vi "Remove Topic.vi"(8 "error in (no error)":errorcluster, 10 "Topic":refnum<class "Topic.lvclass">, 11 "TopicLookupTable":refnum<data-value>) -> (0 "error out":errorcluster, 3 "TopicLookupTable":refnum<data-value>)   [LabVIEW 2017, in "Mediator.lvlib" / "TopicLookupTable.lvclass"]
doc: "<License>\nCopyright © 2017 Composed Systems, LLC | All rights reserved\nwww.composed.io\n\nAuthor: Ethan Stern <ethan.stern@composed.io>\n\nThis software is provided \"AS IS\" WITHOUT WARRANTIES, either express or implied, AND IS FOR EDUCATIONAL PURPOSES ONLY.\n</License>"
uses:
  TopicLookupTable.lvclass
  Topic/Topic.lvclass
  C:/Program Files (x86)/National Instruments/LabVIEW 2017/vi.lib/ActorFramework/Actor/Actor.lvclass
  TopicLookupTable.lvclass/TopicLookupTable.ctl
  <vilib>/ActorFramework/Actor/Actor.lvclass/Actor.ctl
  <vilib>/ActorFramework/Message Enqueuer/Message Enqueuer.lvclass/Message Enqueuer.ctl
  Topic/Topic.lvclass/Topic.ctl
  <vilib>/ActorFramework/Message Enqueuer/Message Enqueuer.lvclass
  <vilib>/ActorFramework/Actor/Read Self Enqueuer.vi
  <vilib>/ActorFramework/Message Enqueuer/Init from Existing Queue.vi
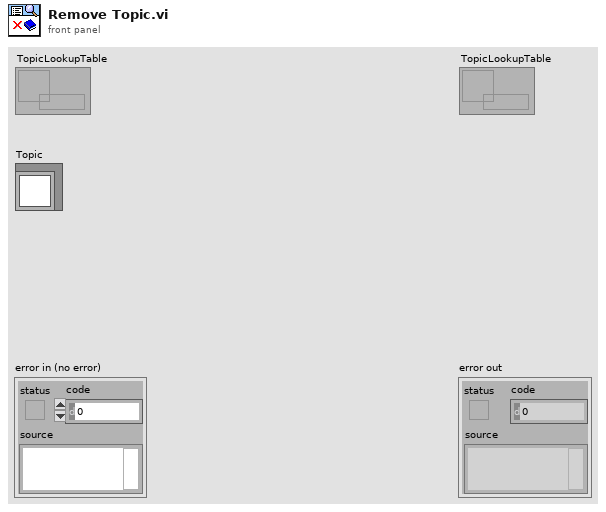
[diagram p1: front panel]
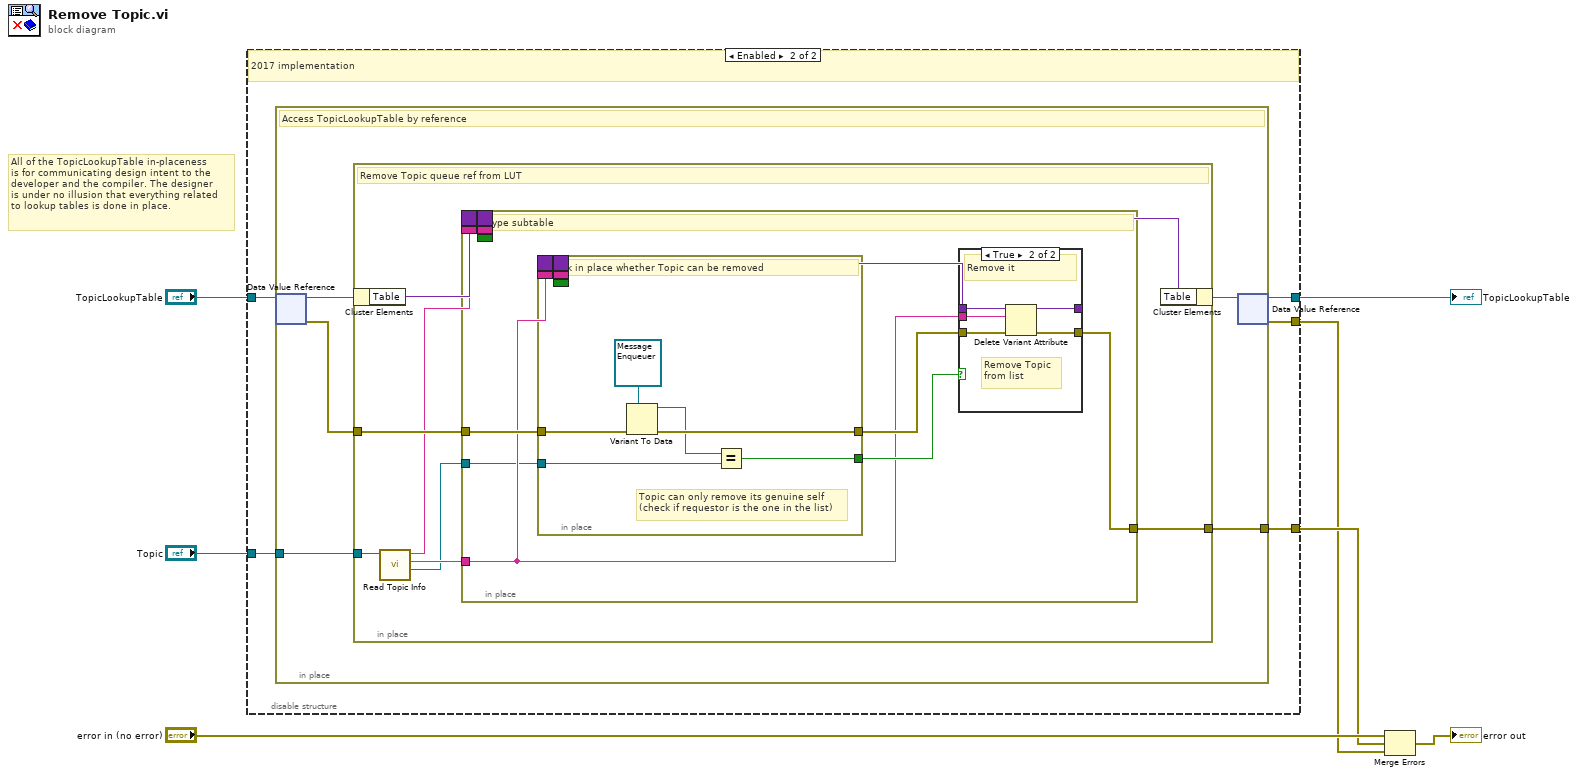
[diagram p0: block diagram]
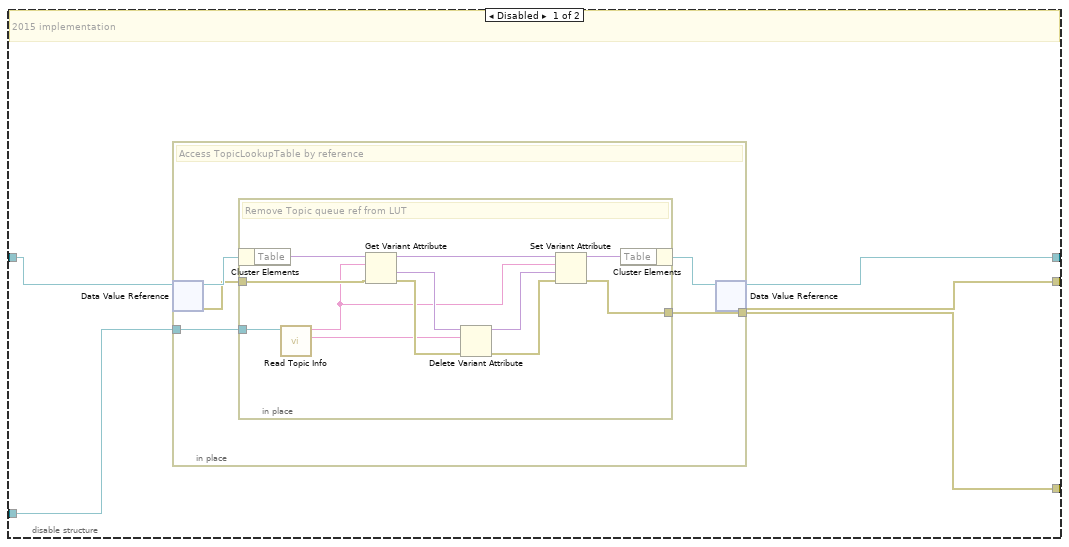
[diagram p2: hidden frame]
diagram:
  # "All of the TopicLookupTable in-placeness\nis for communicating design intent to the\ndeveloper and the compiler. The designer\nis under no illusion that everything related\nto lookup tables is done in place."
  n1 = disable-structure shown="Enabled" {
    disable-tunnel: [w12 w30] -> w5
    disable-tunnel: "Topic" -> [w11 w34]
    disable-tunnel: "TopicLookupTable" -> [w10 w33]
    disable-tunnel: [w9 w32] -> w2
    disable-tunnel: [w8 w31] -> w1
    frame Disabled {
      # "2015 implementation"
      n2 = in-place {
        in-place-border: [w17] -> w12
        in-place-border: w11 -> [w16]
        # "Access TopicLookupTable by reference"
        n3 = in-place-dvr #1(w10) -> (w15:refnum<class "TopicLookupTable.lvclass">, w13:errorcluster)
        n4 = in-place {
          in-place-border: [w26] -> w17
          in-place-border: w16 -> [w18]
          in-place-border: w13 -> [w28]
          # "Remove Topic queue ref from LUT"
          n5 = in-place-cluster #2(w15) -> ("Table"=w25:variant)
          n6 = call "Read Topic Info.vi"("Topic in"=w18) -> ("Name"=w20:string, "Type"=w19:string)  [unwired: 7 in, 2 out]
          n7 = Get Variant Attribute(Variant=w25, name=w19, error in=w28) -> (duplicate Variant=w24:variant, value=w23:variant, error out=w29:errorcluster)  [unwired: 1 in, 1 out]
          n8 = Delete Variant Attribute(4:w29, 6:w20, 7:w23) -> (0:w21:errorcluster, 3:w22:variant)  [unwired: 1 out]
          n9 = Set Variant Attribute(Variant=w24, name=w19, value=w22, error in=w21) -> (Variant out=w27:variant, error out=w26:errorcluster)  [unwired: 1 out]
          n10 = in-place-cluster #2("Table"=w27) -> (w14:refnum<class "TopicLookupTable.lvclass">)
        }
        n11 = in-place-dvr #1(w14) -> (w8:refnum<data-value>, w9:errorcluster)
      }
    }
    frame Enabled {
      # "2017 implementation"
      n12 = in-place {
        in-place-border: w34 -> [w39]
        in-place-border: [w35] -> w30
        # "Access TopicLookupTable by reference"
        n13 = in-place-dvr #3(w33) -> (w38:refnum<class "TopicLookupTable.lvclass">, w36:errorcluster)
        n14 = in-place {
          in-place-border: w39 -> [w44]
          in-place-border: w36 -> [w43]
          in-place-border: [w42] -> w35
          # "Remove Topic queue ref from LUT"
          n15 = in-place-cluster #4(w38) -> ("Table"=w46:variant)
          n16 = call "Read Topic Info.vi"("Topic in"=w44) -> ("Enqueuer (UID)"=w40:refnum<class "Message Enqueuer.lvclass">, "Name"=w47:string, "Type"=w41:string)  [unwired: 7 in, 1 out]
          n17 = in-place {
            in-place-border: w47 -> [w49]
            border: w46 -> [_]
            border: w41 -> [_]
            border: [_] -> w45
            border: _ -> [_]
            border: _ -> [_]
            in-place-border: w43 -> [w55]
            in-place-border: [w50] -> w42
            in-place-border: w40 -> [w48]
            # "Get type subtable"
            n18 = in-place {
              border: w56 -> [_]
              border: w49 -> [_]
              border: [_] -> w54
              border: _ -> [_]
              border: _ -> [_]
              in-place-border: w48 -> [w65]
              in-place-border: w55 -> [w69]
              in-place-border: [w67] -> w51
              in-place-border: [w66] -> w52
              # "Topic can only remove its genuine self\n(check if requestor is the one in the list)"
              # "Check in place whether Topic can be removed"
              n19 = Variant To Data(error in=w69, type=refnum<class "Message Enqueuer.lvclass"> refnum ("Self Enqueuer"), Variant=w68) -> (data=w64:refnum<class "Message Enqueuer.lvclass">, error out=w67:errorcluster)
              n20 = Equal?(x=w64, y=w65) -> (x = y?=w66:bool)
            }
            n21 = case shown="True" w52 {
              tunnel: w54 -> [w57 w63]
              tunnel: [w57 w62] -> w53
              tunnel: w49 -> [_ w61]
              tunnel: w51 -> [w58 w60]
              tunnel: [w58 w59] -> w50
              frame False {
                # "Topic in list is\nnot requestor"
                # "Do not remove"
              }
              frame True {
                # "Remove Topic\nfrom list"
                # "Remove it"
                n22 = Delete Variant Attribute(4:w60, 6:w61, 7:w63) -> (0:w59:errorcluster, 3:w62:variant)  [unwired: 1 out]
              }
            }
          }
          n23 = in-place-cluster #4("Table"=w45) -> (w37:refnum<class "TopicLookupTable.lvclass">)
        }
        n24 = in-place-dvr #3(w37) -> (w31:refnum<data-value>, w32:errorcluster)
      }
    }
  }
  "TopicLookupTable" <- w1
  n25 = Merge Errors("error in (no error)", w5, w2) -> (→"error out":errorcluster)
